vi "AP2x4x DataTransferRead.vi"(5 "Data scale":enum16{"Linear", "Log"}(ring), 6 "Trace number (1-6)":i8, 7 "error in":errorcluster, 10 "AP2x4x IN":refnum<visa-resource-name>="TCPIP0::169.254.53.138::5900::SOCKET") -> (0 "error out":errorcluster, 1 "read buffer":string, 2 "return count":u32, 3 "AP2x4x OUT":refnum<visa-resource-name>="TCPIP0::169.254.53.138::5900::SOCKET")   [LabVIEW 2014]
panel:
  # "Don't forget to specify Y unit in \"AP2x4x ScaleYUnit\" VI"
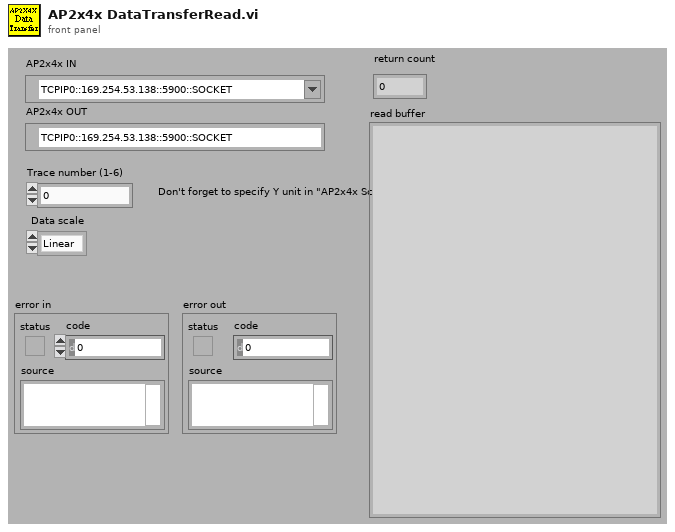
[diagram p1: front panel]
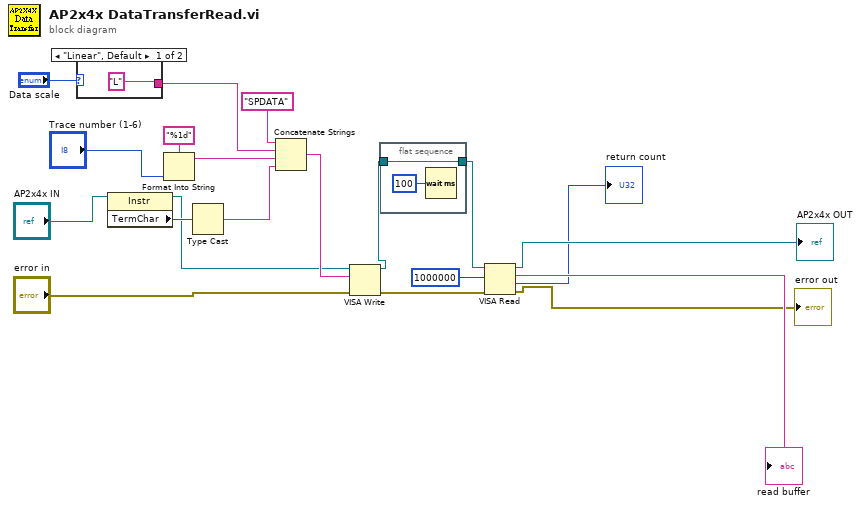
[diagram p0: block diagram]
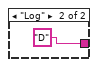
[diagram p2: hidden frame]
diagram:
  n1 = case shown="\"Linear\", Default" "Data scale" {
    tunnel: ["L" "D"] -> w9
    frame "Linear", Default {
    }
    frame "Log" {
    }
  }
  n2 = property class="Instr"(reference="AP2x4x IN") -> (reference out=w15:refnum<visa-resource-name>, "TermChar"=w18:u8)  [unwired: 1 in, 1 out]
  n3 = Format Into String(format string="%1d", "Trace number (1-6)") -> (resulting string=w13:string)  [unwired: 2 in, 1 out]
  n4 = Type Cast(x=w18) -> (*(type *) &x=w16:string)  [unwired: 1 in]
  n5 = Concatenate Strings("SPDATA" ("string"), w9, w13, w16) -> (w19:string)
  n6 = VISA Write(VISA resource name=w15, write buffer=w19, error in (no error)="error in") -> (VISA resource name out=w7:refnum<visa-resource-name>, error out=w6:errorcluster)  [unwired: 1 out]
  n7 = flat-sequence {
    tunnel: w7 -> [w23]
    tunnel: [w23] -> w8
    frame #0 {
      n8 = Wait (ms)(milliseconds to wait=u32 100) -> ()  [unwired: 1 out]
    }
  }
  n9 = VISA Read(VISA resource name=w8, byte count=u32 1000000, error in (no error)=w6) -> (VISA resource name out=→"AP2x4x OUT":refnum<visa-resource-name>, read buffer=→"read buffer":string, return count=→"return count":u32, error out=→"error out":errorcluster)
